vi "Get Execution Units.vi"(8 "error in":errorcluster, 11 "custom device ref":T1 format="%.0x") -> (0 "error out":errorcluster, 1 "List of Execution Units":string[](array[string]), 2 "Execution Units Refs":T1[](array[typedef]) format="%.0x", 3 "custom device ref out":T1 format="%.0x")   [LabVIEW 2020, in "AIM ARINC 664 Scripting.lvlib"]
uses:
  AIM ARINC 664 Scripting.lvlib
  <vilib>/NI VeriStand/Custom Device API/Custom Device Item Ref.ctl
  <vilib>/NI VeriStand/Custom Device API/Custom Device API.lvlib
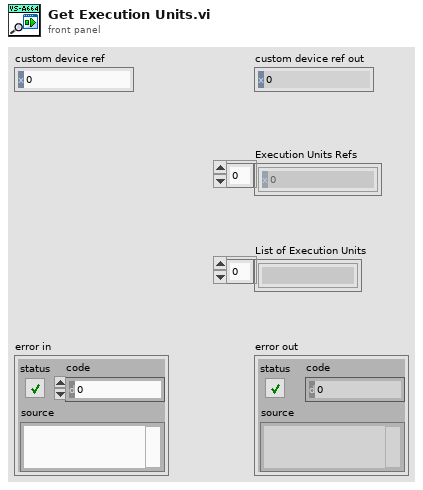
[diagram p1: front panel]
types:
  T1 = typedef "Custom Device API.lvlib/Custom Device Item Ref.ctl" = u64
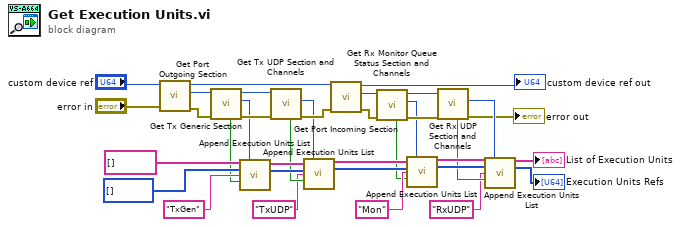
[diagram p0: block diagram]
diagram:
  n1 = call "Get Port Outgoing Section.vi"("error in"="error in", "ports ref"="custom device ref") -> ("error out"=w33:errorcluster, "outgoing section ref out"=w34:T1, "ports ref out"=w32:T1)  [unwired: 6 in, 1 out]
  n2 = call "Get Tx Generic Section.vi"("error in"=w33, "Parent section Ref in"=w34) -> ("error out"=w22:errorcluster, "Item Ref"=w19:T1, "Parent section Ref out"=w21:T1, "found?"=w20:bool)  [unwired: 6 in]
  n3 = call "Append Execution Units List.vi"("Input List"=string[] [] ("appended array"), "Item Ref"=w19, "Input Refs"=T1[] [] ("appended array"), "Execution Unit Name"="TxGen", "Found?"=w20) -> ("List Out"=w27:string[], "Ref Out"=w26:T1[])  [unwired: 9 in]
  n4 = call "Get Tx UDP Section and Channels.vi"("error in"=w22, "custom device ref in"=w21) -> ("error out"=w16:errorcluster, "Tx UDP section ref out"=w3:T1, "channels found?"=w18:bool)  [unwired: 4 in, 3 out]
  n5 = call "Append Execution Units List.vi"("Input List"=w27, "Item Ref"=w3, "Input Refs"=w26, "Execution Unit Name"="TxUDP", "Found?"=w18) -> ("List Out"=w15:string[], "Ref Out"=w13:T1[])  [unwired: 9 in]
  n6 = call "Get Port Incoming Section.vi"("error in"=w16, "ports ref"=w32) -> ("error out"=w25:errorcluster, "incoming ref out"=w24:T1, "ports ref out"=→"custom device ref out":T1)  [unwired: 6 in, 1 out]
  n7 = call "Get Rx Monitor Queue Status Section and Channels.vi"("error in"=w25, "custom device ref in"=w24) -> ("error out"=w10:errorcluster, "Rx monitor section ref out"=w9:T1, "custom device ref out"=w23:T1, "found?"=w6:bool)  [unwired: 5 in, 1 out]
  n8 = call "Append Execution Units List.vi"("Input List"=w15, "Item Ref"=w9, "Input Refs"=w13, "Execution Unit Name"="Mon", "Found?"=w6) -> ("List Out"=w14:string[], "Ref Out"=w12:T1[])  [unwired: 9 in]
  n9 = call "Get Rx UDP Section and Channels.vi"("error in"=w10, "custom device ref in"=w23) -> ("error out"=→"error out":errorcluster, "Rx UDP section ref out"=w8:T1, "found?"=w5:bool)  [unwired: 5 in, 2 out]
  n10 = call "Append Execution Units List.vi"("Input List"=w14, "Item Ref"=w8, "Input Refs"=w12, "Execution Unit Name"="RxUDP", "Found?"=w5) -> ("List Out"=→"List of Execution Units":string[], "Ref Out"=→"Execution Units Refs":T1[])  [unwired: 9 in]
